vi "Calc Exec Step.vi"(8 "error in (no error)":errorcluster, 11 "Stand in":refnum<class "Stand.lvclass">) -> (0 "error out":errorcluster, 3 "Stand out":refnum<class "Stand.lvclass">)   [LabVIEW 2019, in "Stand.lvclass"]
uses:
  Stand.lvclass
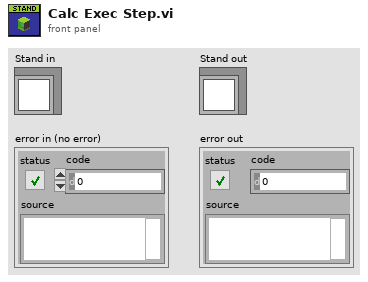
[diagram p1: front panel]
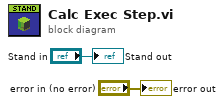
[diagram p0: block diagram]
diagram:
  "Stand out" <- "Stand in"
  "error out" <- "error in (no error)"
